vi "IDS_rt_setAaf.vi"(0 "deviceHandle":i32, 5 "set":i32, 7 "attenuation":i32, 9 "window":i32, 11 "error in (no error)":errorcluster) -> (4 "deviceHandle out":i32, 15 "error out":errorcluster)   [LabVIEW 2016]
doc: "int IDS_DLL IDS_ecu_enable();"
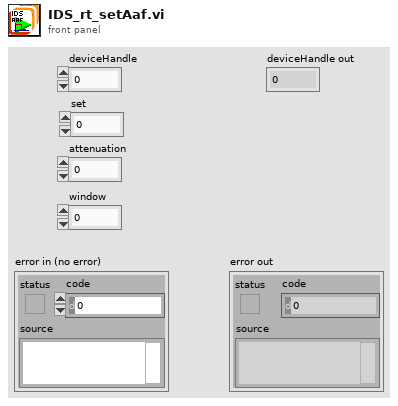
[diagram p1: front panel]
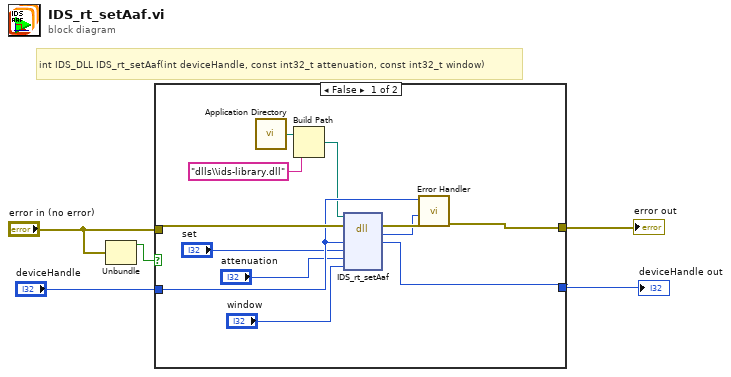
[diagram p0: block diagram]
diagram:
  # "int IDS_DLL IDS_rt_setAaf(int deviceHandle, const int32_t attenuation, const int32_t window)"
  n1 = Unbundle("error in (no error)") -> ("status"=w1:bool)  [unwired: 2 out]
  n2 = case shown="False" w1 {
    tunnel: "error in (no error)" -> [w17 w19]
    tunnel: [w15 w19] -> w5
    tunnel: "deviceHandle" -> [w13 w18]
    tunnel: [w14 w18] -> w3
    frame False {
      n3 = call <vilib>:"Application Directory.vi"() -> ("Application Directory"=w8:path)
      n4 = Build Path(base path=w8, name or relative path="dlls\\ids-library.dll" ("ipAddress")) -> (appended path=w6:path)
      n5 = dll-call lib="C:/Users/matheus/Desktop/LabVIEW_Draft_V1.6.0/dlls/ids-library.*" fn="IDS_rt_setAaf"(path in=w6, error in=w17, "deviceHandle"=w13, "set"="set", "attenuation"="attenuation", "window"="window") -> (error out=w16:errorcluster, "return type"=w12:i32, "deviceHandle"=w14:i32)  [unwired: 4 in, 1 out]
      n6 = call "Error Handler.vi"("error in (no error)"=w16, "error code"=w12, "deviceHandle"=w13) -> ("error out"=w15:errorcluster)  [unwired: 7 in, 1 out]
    }
    frame True {
    }
  }
  "error out" <- w5
  "deviceHandle out" <- w3
